vi "Save Measurement to BD.vi"(8 "error in":errorcluster, 10 "GTron DB":path=path "D:/SQL Database/Gtron Database.db", 11 "Values":string[][](array[string])) -> (0 "error out":errorcluster)   [LabVIEW 2019, in "DataLogger.lvclass"]
doc: "Save Measurement Details"
uses:
  DataLogger.lvclass
  <vilib>/drjdpowell/SQLite Library/SQL Connection/Open (path).vi
  <vilib>/drjdpowell/SQLite Library/SQL Connection/Connection.lvclass
  <vilib>/drjdpowell/SQLite Library/SQL Statement/SQL Statement.lvclass
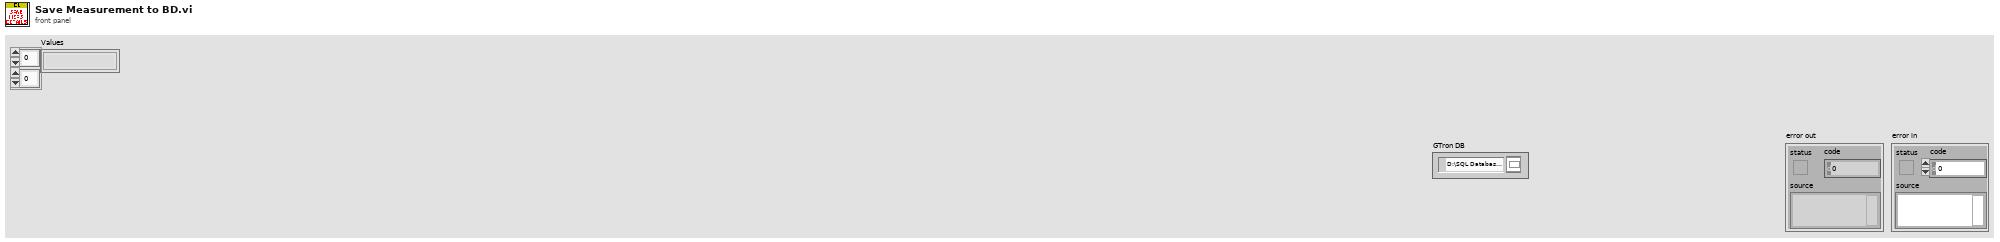
[diagram p1: front panel]
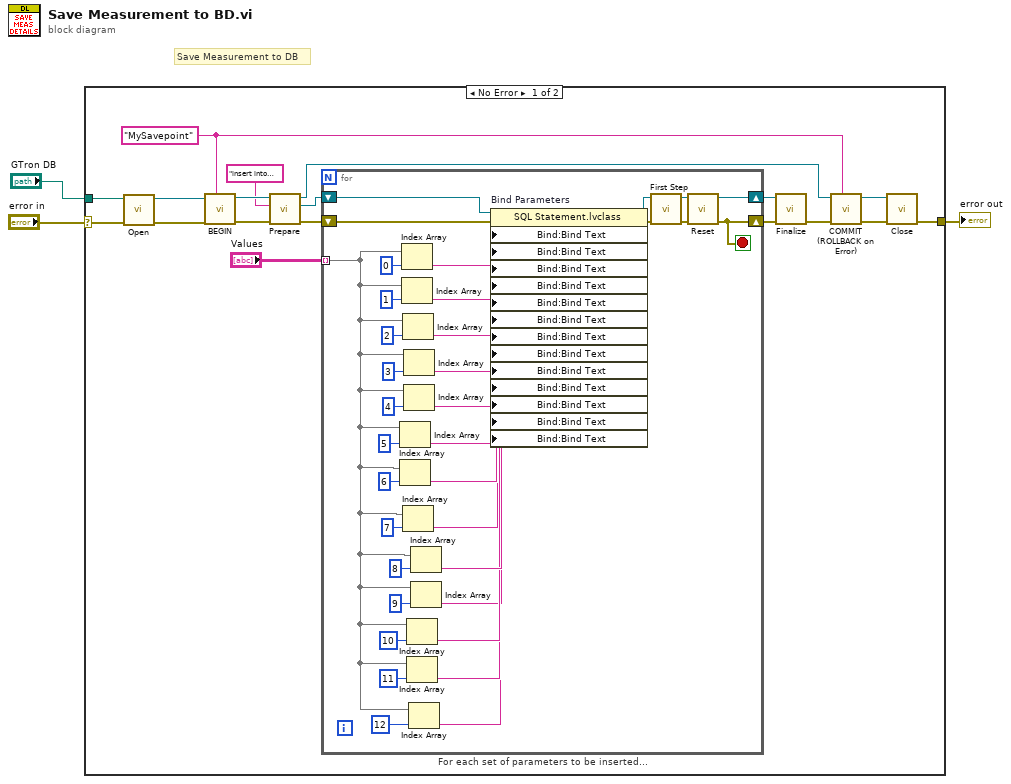
[diagram p0: block diagram]
diagram:
  # "Save Measurement to DB"
  n1 = case shown="No Error" "error in" {
    selector: "error in" -> [w4 w57]
    tunnel: "GTron DB" -> [w10 _]
    tunnel: [w9 w57] -> w2
    frame No Error {
      w13 = "MySavepoint" ("Savepoint name")
      n2 = call-poly <vilib>:"Open.vi"("error in (no error)"=w4, "db file"=w10) -> ("error out"=w21:errorcluster, "SQLite Connection"=w20:refnum<class "Connection.lvclass">)  [unwired: 8 in]
      n3 = call <vilib>:"BEGIN.vi"("Savepoint name"=w13, "error in (no error)"=w21, "Connection in"=w20) -> ("error out"=w14:errorcluster, "Connection out"=w15:refnum<class "Connection.lvclass">)  [unwired: 7 in]
      n4 = call <vilib>:"Prepare.vi"("error in (no error)"=w14, "SQL"="insert into MeasurementDetails  VALUES (?,?,?,?,?,?,?,?,?,?,?,?,?)" ("INSERT statement"), "SQLite Connection in"=w15) -> ("error out"=w18:errorcluster, "SQL Statement"=w19:refnum<class "SQL Statement.lvclass">, "SQLite Connection"=w12:refnum<class "Connection.lvclass">)  [unwired: 4 in, 2 out]
      n5 = for "For each set of parameters to be inserted..." {
        shift-right: [w54] -> w17
        shift-left: w19 -> [w56]
        shift-right: [w53] -> w16
        shift-left: w18 -> [w55]
        tunnel: "Values" -> [w22] mode=indexing
        stop <- w53 stop-if-true
        n6 = Index Array(array=w22, index=5) -> (element=w36:string)
        n7 = Index Array(array=w22, index=6) -> (element=w35:string)
        n8 = Index Array(array=w22, index=0) -> (element=w41:string)
        n9 = Index Array(array=w22, index=1) -> (element=w40:string)
        n10 = Index Array(array=w22, index=2) -> (element=w39:string)
        n11 = Index Array(array=w22, index=7) -> (element=w33:string)
        n12 = Index Array(array=w22, index=3) -> (element=w38:string)
        n13 = Index Array(array=w22, index=4) -> (element=w37:string)
        n14 = Index Array(array=w22, index=10) -> (element=w28:string)
        n15 = Index Array(array=w22, index=11) -> (element=w27:string)
        n16 = Index Array(array=w22, index=12) -> (element=w23:string)
        n17 = Index Array(array=w22, index=8) -> (element=w29:string)
        n18 = Index Array(array=w22, index=9) -> (element=w26:string)
        n19 = property on="Bind Parameters" class="SQL Statement.lvclass"(reference=w56, error in=w55, "Bind:Bind Text"=w41, "Bind:Bind Text"=w40, "Bind:Bind Text"=w39, "Bind:Bind Text"=w38, "Bind:Bind Text"=w37, "Bind:Bind Text"=w36, "Bind:Bind Text"=w35, "Bind:Bind Text"=w33, "Bind:Bind Text"=w29, "Bind:Bind Text"=w26, "Bind:Bind Text"=w28, "Bind:Bind Text"=w27, "Bind:Bind Text"=w23) -> (reference out=w52:refnum<class "SQL Statement.lvclass">, error out=w51:errorcluster)
        n20 = call <vilib>:"First Step.vi"("error in (no error)"=w51, "SQL Statement in"=w52) -> ("error out"=w50:errorcluster, "SQL Statement"=w49:refnum<class "SQL Statement.lvclass">)  [unwired: 7 in, 1 out]
        n21 = call <vilib>:"Reset.vi"("error in (no error)"=w50, "SQL Statement in"=w49) -> ("error out"=w53:errorcluster, "SQL Statement"=w54:refnum<class "SQL Statement.lvclass">)  [unwired: 8 in]
      }
      n22 = call <vilib>:"Finalize.vi"("error in (no error)"=w16, "SQL Statement in"=w17) -> ("error out"=w11:errorcluster)  [unwired: 9 in]
      n23 = call <vilib>:"COMMIT (ROLLBACK on Error).vi"("Savepoint name"=w13, "error in (no error)"=w11, "Connection in"=w12) -> ("error out"=w7:errorcluster, "Connection out"=w8:refnum<class "Connection.lvclass">)  [unwired: 7 in]
      n24 = call-dynamic "Close.vi"("error in (no error)"=w7, "SQLite Connection in"=w8) -> ("error out"=w9:errorcluster)  [unwired: 9 in]
    }
    frame Error {
    }
  }
  "error out" <- w2
